vi "Connect.vi"(0 "reference in":refnum<class "Simulated-PowerModule.lvclass">, 11 "Error In":errorcluster) -> (4 "reference out":refnum<class "Simulated-PowerModule.lvclass">, 15 "Error Out":errorcluster)   [LabVIEW 2023, in "Simulated-PowerModule.lvlib" / "Simulated-PowerModule.lvclass"]
uses:
  Simulated-PowerModule.lvclass
  Simulated-PowerModule.lvclass/Simulated-PowerModule.ctl
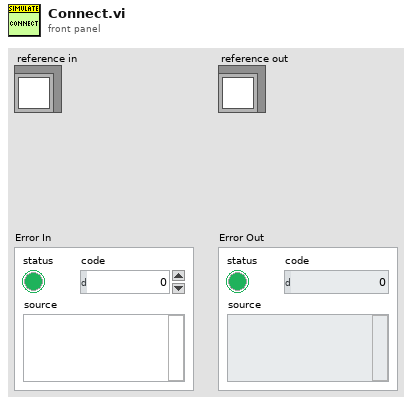
[diagram p1: front panel]
types:
  T1 = typedef "Simulated-PowerModule.lvlib/Simulated-PowerModule.lvclass/ObjectAttributes.ctl" = cluster{"JSON Config Path":path, "Configuration":T2, "connected":bool, "reserved":bool, "setpoint":cluster{"voltage":sgl, "current":sgl, "resistance":sgl}, "last timestamp":i64, "mode":T4, "range":T3, "measurement array":T5[]}
  T2 = typedef "Simulated-PowerModule.lvlib/Simulated-PowerModule.lvclass/Configuration.ctl" = cluster{"range":T3}
  T3 = typedef "PowerModuleInterface.lvlibp/PowerModuleInterface.lvclass/Range.ctl" = cluster{"Current Max (A)":dbl, "Current Min (A)":dbl, "Voltage Max (V)":dbl, "Voltage Min (V)":dbl}
  T4 = typedef "Simulated-PowerModule.lvlib/Simulated-PowerModule.lvclass/Mode.ctl" = u16
  T5 = typedef "PowerModuleInterface.lvlibp/PowerModuleInterface.lvclass/Measurements.ctl" = cluster{"measured voltage (V)":dbl, "measured current (A)":dbl, "setpoint voltage (V)":dbl, "setpoint current (A)":dbl, "timestamp":dbl}
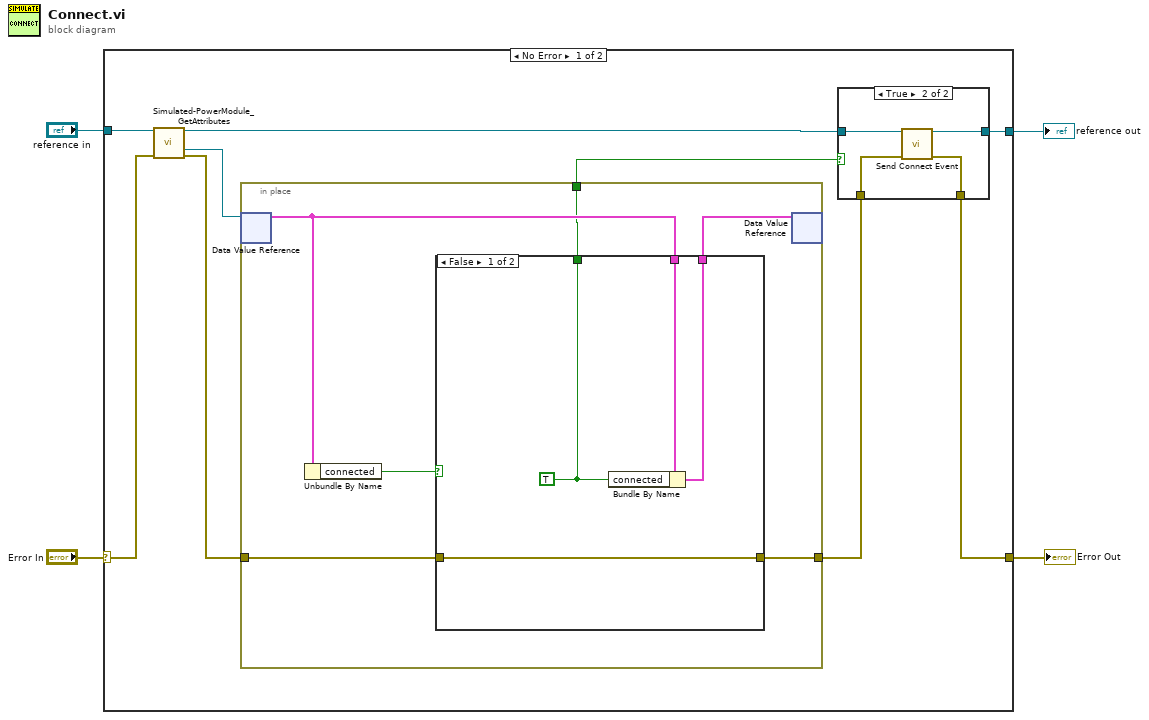
[diagram p0: block diagram]
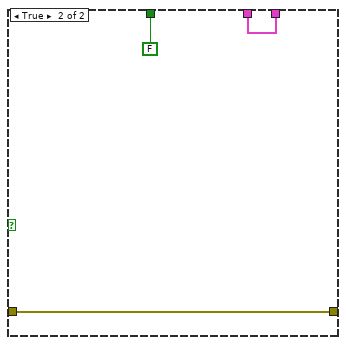
[diagram p2: hidden frame]
diagram:
  n1 = case shown="No Error" "Error In" {
    selector: "Error In" -> [w12 w33]
    tunnel: "reference in" -> [w13 w34]
    tunnel: [w6 w34] -> w2
    tunnel: [w7 w33] -> w1
    frame No Error {
      n2 = call "Simulated-PowerModule_GetAttributes.vi"("reference in"=w13, "Error In"=w12) -> ("reference out"=w9:refnum<class "Simulated-PowerModule.lvclass">, "DataRef"=w11:refnum<data-value>, "Error Out"=w10:errorcluster)  [unwired: 10 in, 1 out]
      n3 = in-place {
        in-place-border: w10 -> [w17]
        in-place-border: [w16] -> w8
        in-place-border: [w15] -> w5
        n4 = in-place-dvr #1(w11) -> (w18:T1)  [unwired: 1 out]
        n5 = Unbundle By Name(w18) -> ("connected"=w14:bool)
        n6 = case shown="False" w14 {
          tunnel: [w23 w26] -> w19
          tunnel: w18 -> [w22 w26]
          tunnel: w17 -> [w20 w24]
          tunnel: [w20 w24] -> w16
          tunnel: [w21 FALSE] -> w15
          frame False {
            w21 = TRUE ("connected")
            n7 = Bundle By Name(cluster=w22, "connected"=w21) -> (w23:T1)
          }
          frame True {
          }
        }
        n8 = in-place-dvr #1(w19) -> ()  [unwired: 2 out]
      }
      n9 = case shown="True" w5 {
        tunnel: w9 -> [w27 w32]
        tunnel: w8 -> [w28 w31]
        tunnel: [w28 w30] -> w7
        tunnel: [w27 w29] -> w6
        frame False {
        }
        frame True {
          n10 = call "Send Connect Event.vi"("reference in"=w32, "Error In"=w31) -> ("reference out"=w29:refnum<class "Simulated-PowerModule.lvclass">, "Error Out"=w30:errorcluster)  [unwired: 12 in]
        }
      }
    }
    frame Error {
    }
  }
  "Error Out" <- w1
  "reference out" <- w2
